vi "Configure Acquisition Record.vi"(0 "VISA Resource Name":refnum<visa-resource-name>, 5 "Time Per Record (1.0e-3 s)":dbl=0.001 format="%^.2e", 7 "Minimum Record Length (2000)":i32=2000, 9 "Acquisition Start Time (0.0 s)":dbl format="%^.2e", 11 "error in (no error)":errorcluster {"code" format="%.0x"}) -> (4 "VISA Resource Name Out":refnum<visa-resource-name>, 15 "error out":errorcluster {"code" format="%.0x"})   [LabVIEW 2011, in "Agilent 546XX Series.lvlib"]
doc: "This VI configures the common properties of the acquisition subsystem. These properties are the time per record, minimum record length, and acquisition start time."
uses:
  Agilent 546XX Series.lvlib
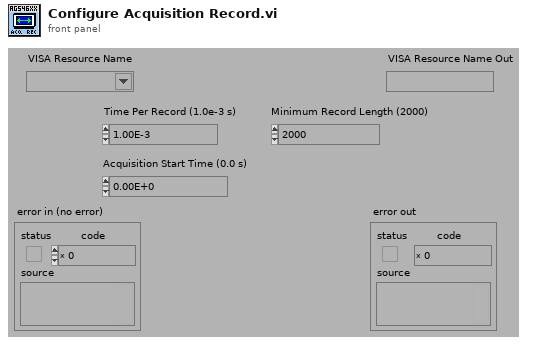
[diagram p1: front panel]
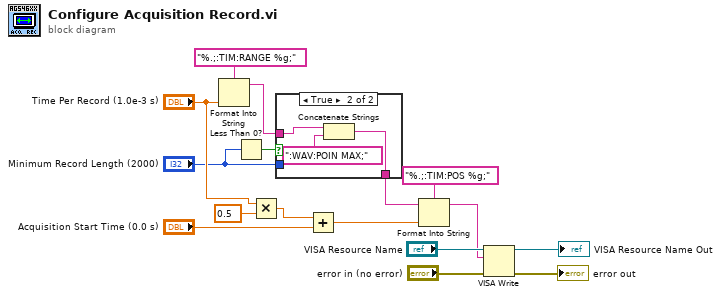
[diagram p0: block diagram]
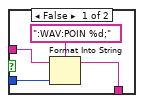
[diagram p2: hidden frame]
diagram:
  n1 = Format Into String(format string="%.;:TIM:RANGE %g;", "Time Per Record (1.0e-3 s)") -> (resulting string=w9:string)  [unwired: 2 in, 1 out]
  n2 = Less Than 0?(x="Minimum Record Length (2000)") -> (x < 0?=w2:bool)
  n3 = Multiply(x="Time Per Record (1.0e-3 s)", y=0.5) -> (x*y=w5:dbl)
  n4 = case shown="True" w2 {
    tunnel: "Minimum Record Length (2000)" -> [w20 _]
    tunnel: w9 -> [w18 w23]
    tunnel: [w17 w21] -> w8
    frame False {
      n5 = Format Into String(format string=":WAV:POIN %d;", initial string=w18, w20) -> (resulting string=w17:string)  [unwired: 1 in, 1 out]
    }
    frame True {
      n6 = Concatenate Strings(w23, ":WAV:POIN MAX;") -> (w21:string)
    }
  }
  n7 = Add(x=w5, y="Acquisition Start Time (0.0 s)") -> (x+y=w7:dbl)
  n8 = Format Into String(format string="%.;:TIM:POS %g;", initial string=w8, w7) -> (resulting string=w10:string)  [unwired: 1 in, 1 out]
  n9 = VISA Write(VISA resource name="VISA Resource Name", write buffer=w10, error in (no error)="error in (no error)") -> (VISA resource name out=→"VISA Resource Name Out":refnum<visa-resource-name>, error out=→"error out":errorcluster)  [unwired: 1 out]
